vi "Arrays 2.vi"() -> ()   [LabVIEW 2014]
panel:
  out "Square Root":dbl[](array[numeric])
  in  "Input Array":dbl[](array[numeric])
  # "Arrays- Second VI"
  # "Input Array"
  # "Square Root"
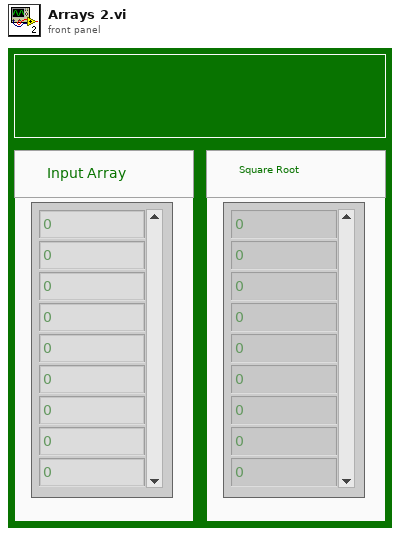
[diagram p1: front panel]
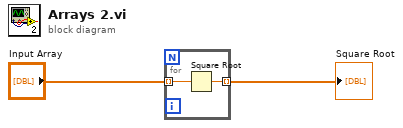
[diagram p0: block diagram]
diagram:
  n1 = for {
    tunnel: "Input Array" -> [w4] mode=indexing
    tunnel: [w3] -> w2 mode=indexing
    n2 = Square Root(x=w4) -> (sqrt(x)=w3:dbl)
  }
  "Square Root" <- w2
